vi "SENDATA.vi"(6 "DATO":string, 8 "error in (no error)":errorcluster, 9 "PROVIENE DE?":enum16{"CONTADOR", "GENERADOR F"}(ring), 10 "Path":path, 11 "GUARDAR_CSV in":refnum<class "GUARDAR_CSV.lvclass">) -> (0 "error out":errorcluster, 3 "GUARDAR_CSV out":refnum<class "GUARDAR_CSV.lvclass">)   [LabVIEW 2019, in "GUARDAR_CSV.lvlib" / "GUARDAR_CSV.lvclass"]
uses:
  GUARDAR_CSV.lvclass
  GUARDAR_CSV.lvclass/GUARDAR_CSV.ctl
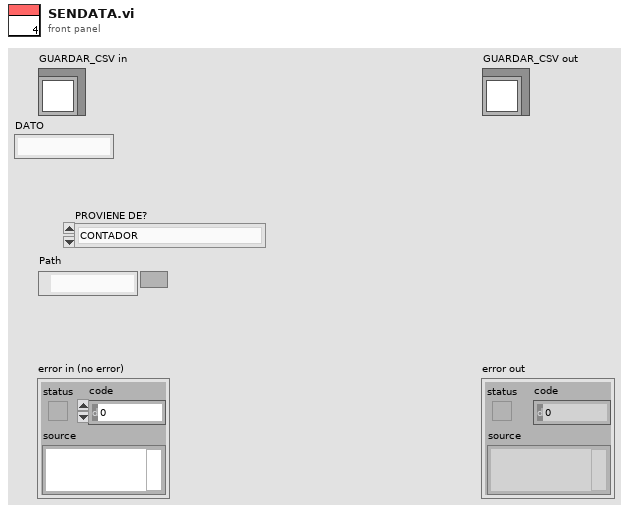
[diagram p1: front panel]
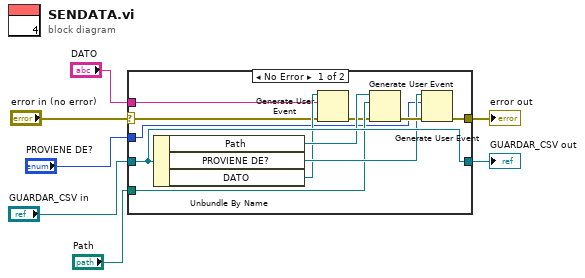
[diagram p0: block diagram]
diagram:
  n1 = case shown="No Error" "error in (no error)" {
    selector: "error in (no error)" -> [w10 w20]
    tunnel: [w9 w20] -> w6
    tunnel: [w17 w19] -> w4
    tunnel: "GUARDAR_CSV in" -> [w17 w19]
    tunnel: "DATO" -> [w13 _]
    tunnel: "Path" -> [w12 _]
    tunnel: "PROVIENE DE?" -> [w8 _]
    frame No Error {
      n2 = Unbundle By Name(w17) -> ("Path"=w16:refnum<user-event>, "PROVIENE DE?"=w15:refnum<user-event>, "DATO"=w14:refnum<user-event>)
      n3 = Generate User Event(user event=w14, event data cluster=w13, error in=w10) -> (error out=w11:errorcluster)  [unwired: 1 in, 1 out]
      n4 = Generate User Event(user event=w16, event data cluster=w12, error in=w11) -> (error out=w18:errorcluster)  [unwired: 1 in, 1 out]
      n5 = Generate User Event(user event=w15, event data cluster=w8, error in=w18) -> (error out=w9:errorcluster)  [unwired: 1 in, 1 out]
    }
    frame Error {
    }
  }
  "error out" <- w6
  "GUARDAR_CSV out" <- w4
